vi "M Power Plant.vi"(11 "EV3 in":T1) -> ()   [LabVIEW 2016]
uses:
  <vilib>/NXT/Subs/LVHSConnector.ctl
  <vilib>/NXT/LegoClasses/BrickReference/BrickReference.lvclass
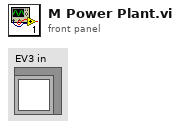
[diagram p1: front panel]
types:
  T1 = typedef "LVHSConnector.ctl" = refnum<class "BrickReference.lvclass">
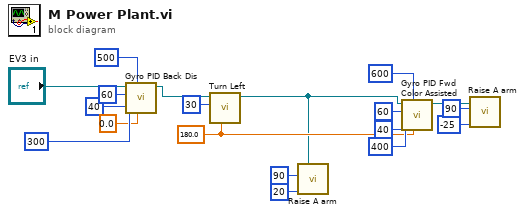
[diagram p0: block diagram]
diagram:
  w7 = sgl 180.0 ("Turning angle")
  n1 = call "Gyro PID Back Dis.vi"("Target angle"=sgl 0.0, "Threshold to stop"=500, "Threshold to slow"=300, "Min. speed"=40, "Max. speed"=60, "EV3 in"="EV3 in") -> ("EV3 out"=w13:T1)  [unwired: 5 in]
  n2 = call "Turn Left.vi"("Turning angle"=w7, "Motor B (right)"=i8 30, "EV3 in"=w13) -> ("EV3 out"=w4:T1)  [unwired: 8 in]
  n3 = call "Raise A arm.vi"("Power"=i8 20, "Rotation"=90, "EV3 in"=w4) -> ()  [unwired: 8 in, 1 out]
  n4 = call "Gyro PID Fwd Color Assisted.vi"("Target angle"=w7, "Threshold to Color"=600, "Threshold to slow"=400, "Min. speed"=40, "Max. speed"=60, "EV3 in"=w4) -> ("EV3 out"=w3:T1)  [unwired: 5 in]
  n5 = call "Raise A arm.vi"("Power"=i8 -25, "Rotation"=90, "EV3 in"=w3) -> ()  [unwired: 8 in, 1 out]
